vi "Modbus_FSM_Power_Dependence_Control.vi"() -> ()   [LabVIEW 2021]
uses:
  <vilib>/Plasmionique/MB Master/MB_Master/MB_Master.lvclass
  <vilib>/Plasmionique/MB Master/MB_Master_Serial/MB_Master_Serial.lvclass
  <vilib>/Plasmionique/MB Master/MB Master.lvlib
  <vilib>/Plasmionique/MB Master/MB_ADU/MB_ADU.lvclass
  C:/Program Files/National Instruments/LabVIEW 2021/vi.lib/Plasmionique/MB Master/MB_Master/MB_Master.lvclass
  Camera_Selected_g1.ctl
panel:
  in  "Direction Pulsed":bool
  in  "Total Scan Steps":i32(slide)=1 min=0 max=650000 step=10 scale=1.0..400000.0
  in  "Move Stage":bool
  in  "Scan g(1)":bool
  in  "Direction Stage":bool
  in  "Camera Selected":T1
  out "Scan Segments":i32
  out "Initial Segments":u16=10214
  in  "Steps":i32(slide)=1 min=0 max=650000 step=10 scale=1.0..400000.0
  out "Full Excitation Scan?":bool=TRUE
  out "Current Excitation HWP Segments":u8=230
  out "Initial Excitation QWP Segments":u8
  out "Current Excitation\nQWP angle":sgl
  in  "Event Registration Refnum":refnum<event-registration>
  in  "stop":bool
  out "Reset Modbus?":bool=TRUE
  in  "Modbus Address":refnum<visa-resource-name>="COM21"
  in  "Pulsed Power":dbl(slide)=1.0 min=0.0 max=180.0 step=0.001 scale=0.0..180.0
  in  "Scan Angle \nCW HWP":dbl=45.0
  in  "Etalon Angle":dbl(slide)=1.0 min=0.0 max=180.0 step=0.001 scale=0.0..180.0
  in  "CW Power":dbl(slide)=1.0 min=0.0 max=180.0 step=0.1 scale=0.0..180.0
  in  "Scan Angle\nPulsed HWP":dbl=45.0
  out "Def Pos CH3":u16[](array[numeric])
  out "Def Pos CH2":u16[](array[numeric])
  out "Def Pos CH1":u16[](array[numeric])
  out "Def Pos CH0":u16[](array[numeric])
  in  "Direction Etalon":bool
  in  "Direction CW":bool
  out "CH1 Steps/deg":u16=400
  out "CH0 Steps/deg":u16=400
  out "Current Collection HWP Segments":u8
  out "Initial Pulsed Segments":u8=230
  out "CH2 Steps/deg":u16=400
  out "CH3 Steps/deg":u16=400
  out "Current CW Segments":u8
  out "Initial Collection QWP Segments":u8=230
  out "Current CW angle":sgl
  out "Current Pulsed angle":sgl
  out "Full Collection Scan?":bool=TRUE
  out "Current Pulsed Segments":u8
  out "Initial CW Segments":u8=230
  out "Current Excitation\nHWP angle":sgl
  out "Def Pos CH0 Ind":bool=TRUE
  out "Def Pos CH1 Ind":bool=TRUE
  out "Def Pos CH2 Ind":bool=TRUE
  out "Def Pos CH3 Ind":bool=TRUE
  out "Pulsed?":bool=TRUE
  out "Last RX":string
  out "Last TX":string
  out "Last RX Time":string
  out "dt (ms)":u32=4
  out "Open?":bool
  out "Last Error Time":string
  out "Last Error Status":errorcluster
  in  "Reset Motor":bool
  in  "Rotate Etalon":bool
  in  "CW Power Rotate":bool
  in  "Pulsed Power Rotate":bool
  in  "Absolute Move CH0":bool=TRUE caption="Move to Default"
  in  "Absolute Move CH1":bool=TRUE
  in  "Absolute Move CH2":bool=TRUE
  in  "Absolute Move CH3":bool=TRUE
  in  "Set CH0 Default Position":bool=TRUE caption="Set Default"
  in  "Set CH1 Default Position":bool=TRUE
  in  "Set CH2 Default Position":bool=TRUE
  in  "Set CH3 Default Position":bool=TRUE
  in  "Power Dependence - CW":bool
  in  "Power Dependence - Pulsed":bool
  # "Power"
  # "Power Dependence"
  # "Direction"
  # "Rotate"
  # "g(1)"
  # "Direction"
  # "Etalon"
  # "Direction"
  # "Rotate"
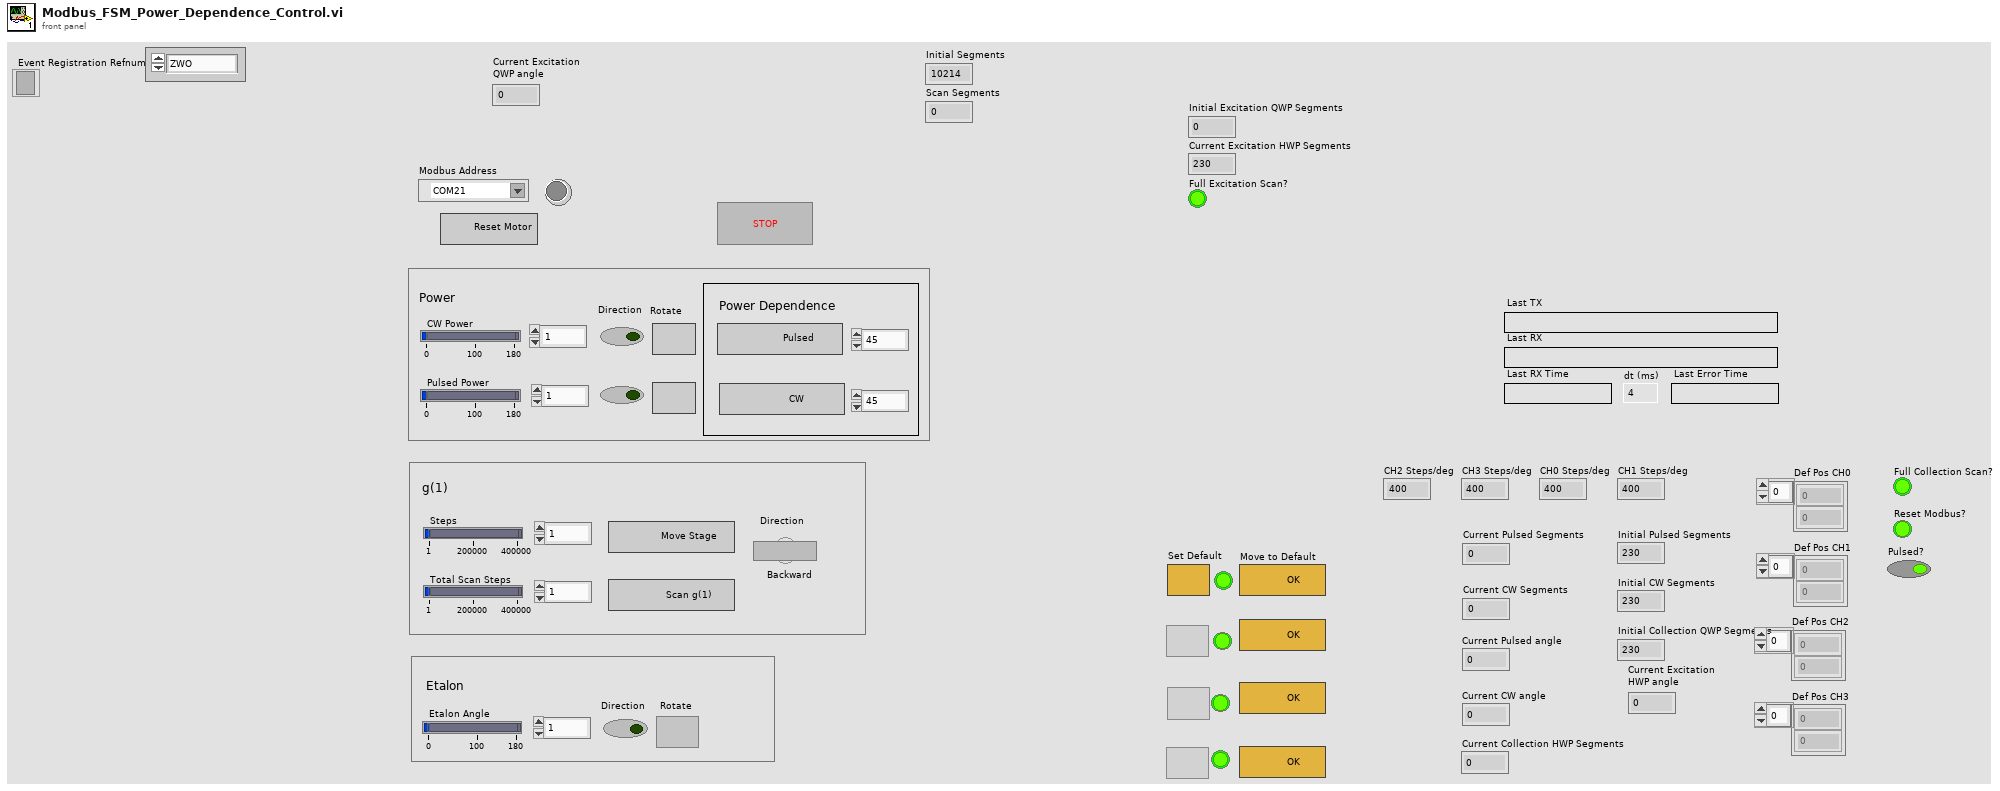
[diagram p1: front panel]
types:
  T1 = typedef "Camera_Selected_g1.ctl" = enum16{"ZWO", "qcmos"}
  T2 = cluster{"baud rate (bps)":u32, "stop bits":u16, "parity":u16, "flow control":u16, "timeout":u32, "retries":i32}
  T3 = enum8{"Enabled", "Disabled", "Disabled and Grayed Out"}
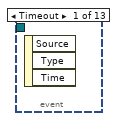
[diagram p2: hidden frame]
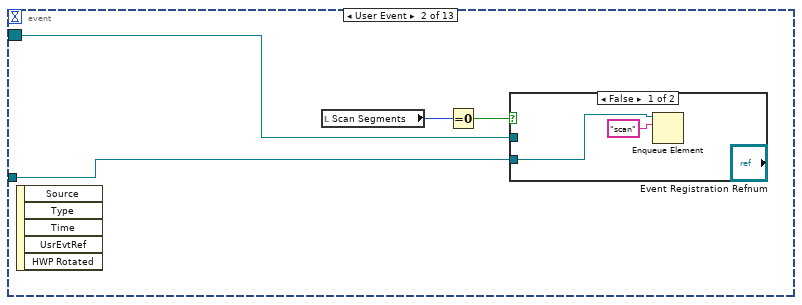
[diagram p3: hidden frame]
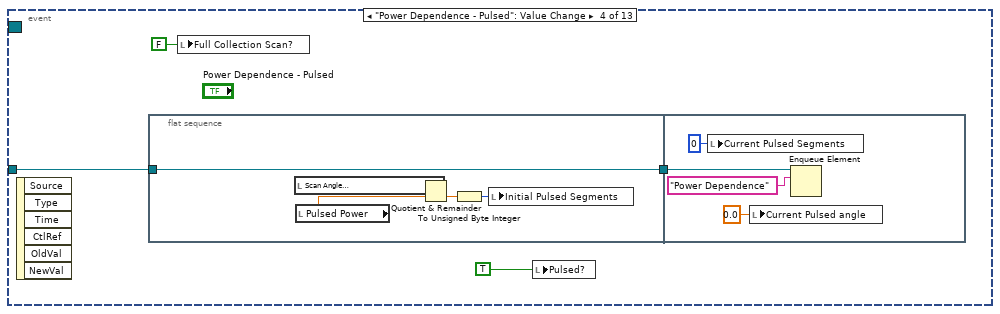
[diagram p5: hidden frame]
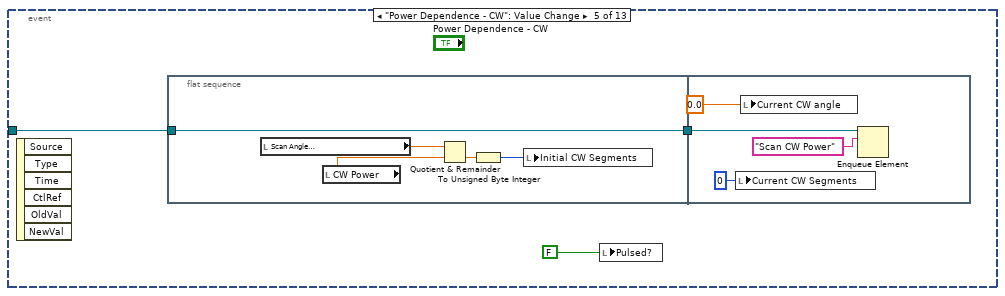
[diagram p6: hidden frame]
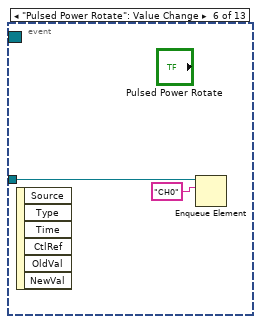
[diagram p7: hidden frame]
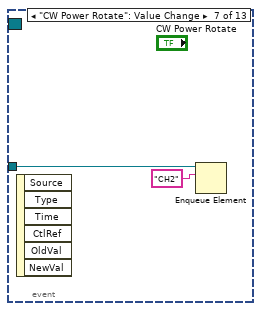
[diagram p8: hidden frame]
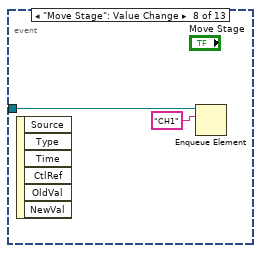
[diagram p9: hidden frame]
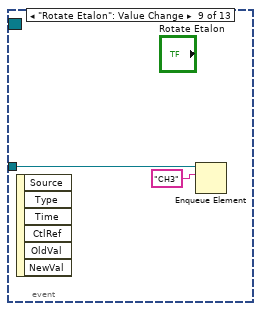
[diagram p10: hidden frame]
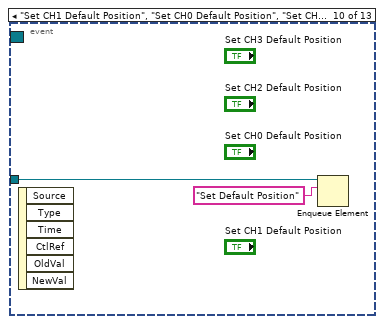
[diagram p11: hidden frame]
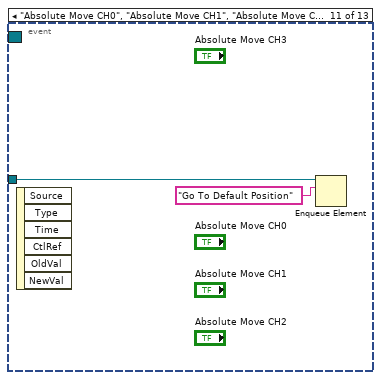
[diagram p12: hidden frame]
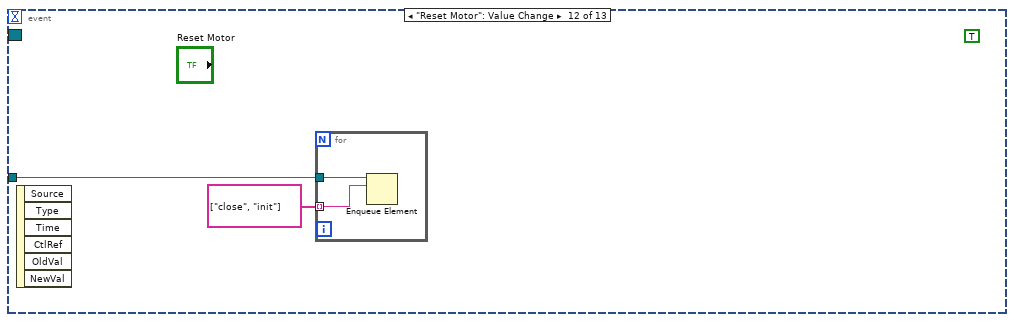
[diagram p13: hidden frame]
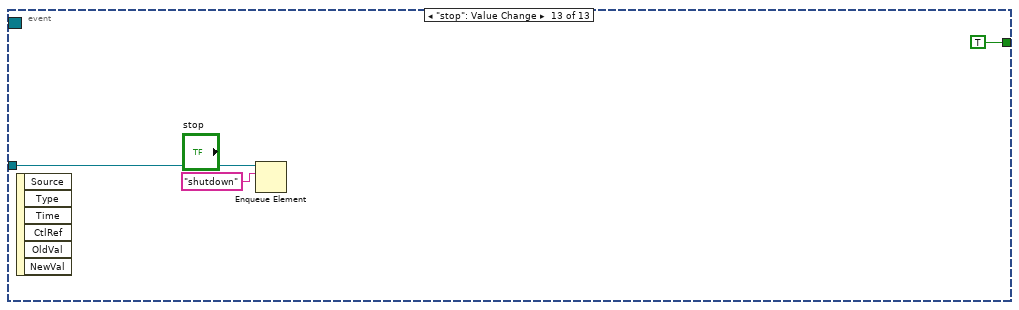
[diagram p14: hidden frame]
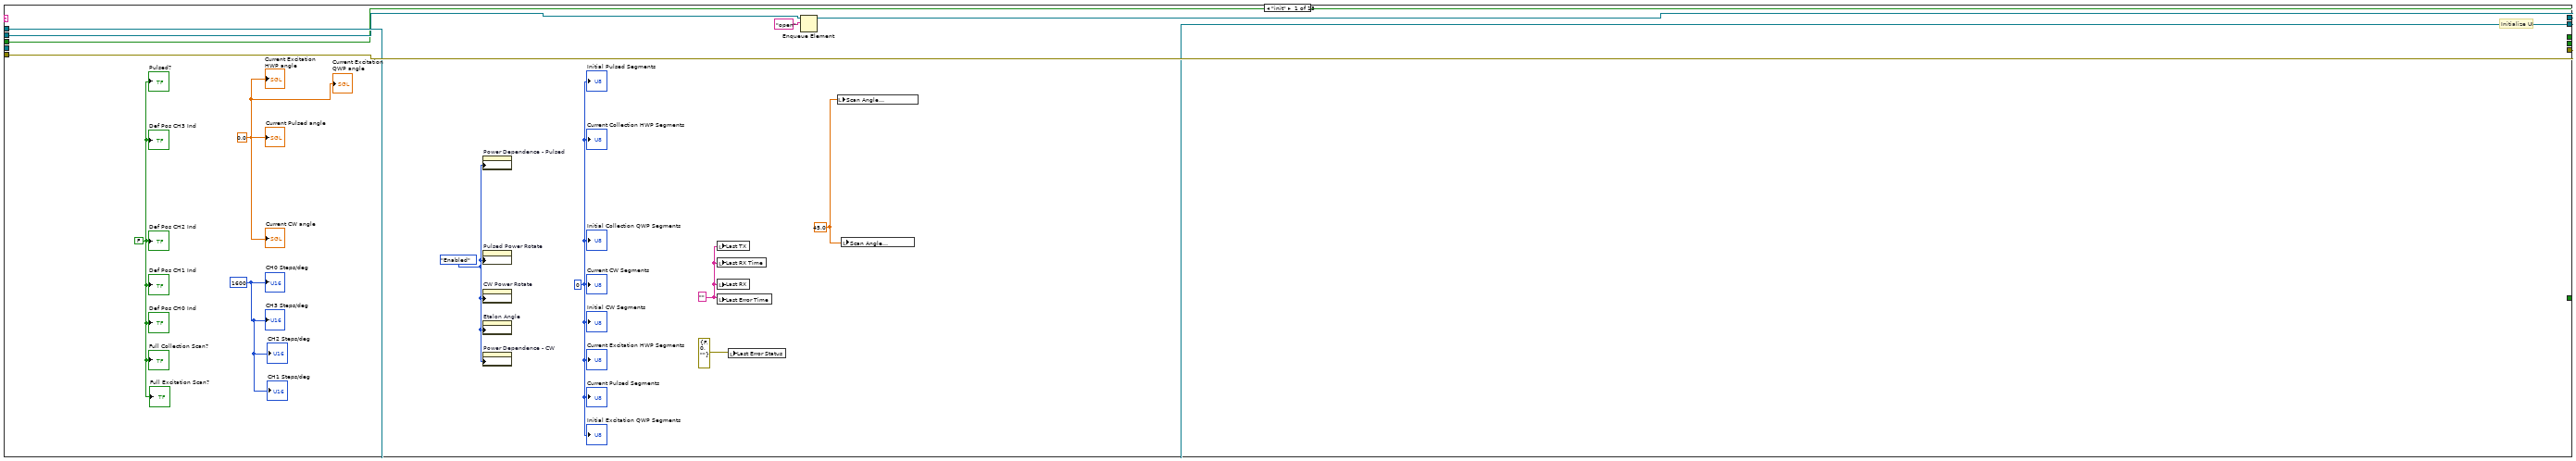
[diagram p17: hidden frame]
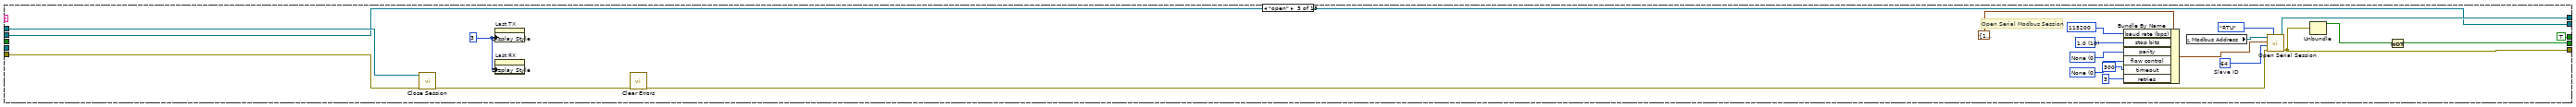
[diagram p18: hidden frame]
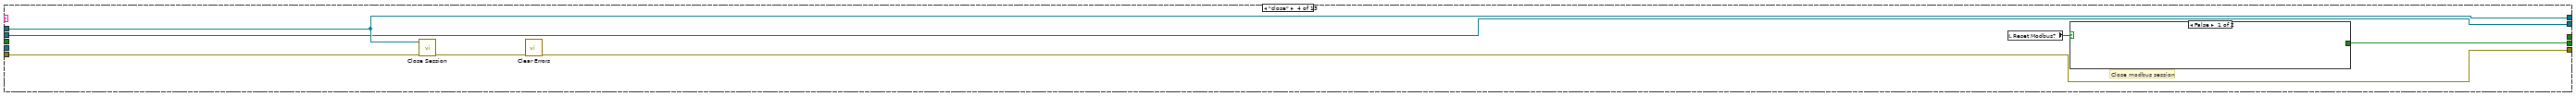
[diagram p19: hidden frame]
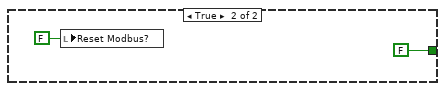
[diagram p20: hidden frame]
diagram:
  w1 = refnum<event-registration> refnum  # Event Registration Refnum
  w2 = refnum<user-event> refnum  # user event out
  n1 = Obtain Queue(element data type="") -> (queue out=w6:refnum<queue>)  [unwired: 4 in, 2 out]
  n2 = Enqueue Element(queue=w6, element="init") -> (queue out=w3:refnum<queue>)  [unwired: 2 in, 2 out]
  n3 = while {
    tunnel: w3 -> [w9]
    tunnel: w1 -> [w7]
    stop <- w8 stop-if-true
    # "UI Event Handler"
    n4 = event shown="[2] \"Scan g(1)\": Value Change" {
      selector: w7 -> [_ w11 _ _ _ _ _ _ _ _ _ _ _]
      dyn-events: _ -> [_ _ _ _ _ _ _ _ _ _ _ _ _]
      timeout: _ -> [_ _ _ _ _ _ _ _ _ _ _ _ _]
      tunnel: w9 -> [_ w10 w16 w25 w37 w48 w50 w52 w54 w55 w57 w60 w63]
      tunnel: [_ _ _ _ _ _ _ _ _ _ _ _ TRUE] -> w8
      event Timeout {
        n5 = event-data() -> ()  [unwired: 1 in, 3 out]
      }
      event User Event {
        n6 = event-data() -> ()  [unwired: 1 in, 5 out]
        n7 = local read "Scan Segments"() -> (w13:i32)
        n8 = Equal To 0?(x=w13) -> (x = 0?=w12:bool)
        n9 = case shown="False" w12 {
          tunnel: w11 -> [_ _]
          tunnel: w10 -> [w14 _]
          frame False {
            n10 = Enqueue Element(queue=w14, element="scan") -> ()  [unwired: 2 in, 3 out]
          }
          frame True {
          }
        }
      }
      event "Scan g(1)": Value Change {
        n11 = event-data() -> ()  [unwired: 1 in, 6 out]
        n12 = flat-sequence {
          tunnel: w16 -> [w20]
          frame #0 {
            n13 = local read "Total Scan Steps"() -> (w17:i32)
            n14 = local read "Steps"() -> (w18:i32)
            n15 = Quotient & Remainder(x=w17, y=w18) -> (floor(x/y)=w19:i32)  [unwired: 1 out]
            n16 = local write "Initial Segments"(w19) -> ()
            n17 = local write "Scan Segments"(w19) -> ()
          }
          frame #1 {
            n18 = Enqueue Element(queue=w20, element="scan") -> ()  [unwired: 2 in, 3 out]
          }
        }
      }
      event "Power Dependence - Pulsed": Value Change {
        n19 = event-data() -> ()  [unwired: 1 in, 6 out]
        n20 = flat-sequence {
          tunnel: w25 -> [w30]
          tunnel: [w30] -> w24
          tunnel: w24 -> [w33]
          frame #0 {
            n21 = local read "Scan Angle\nPulsed HWP"() -> (w26:dbl)
            n22 = local read "Pulsed Power"() -> (w29:dbl)
            n23 = Quotient & Remainder(x=w26, y=w29) -> (floor(x/y)=w28:dbl)  [unwired: 1 out]
            n24 = To Unsigned Byte Integer(number=w28) -> (unsigned 8bit integer=w27:u8)
            n25 = local write "Initial Pulsed Segments"(w27) -> ()
          }
          frame #1 {
            n26 = local write "Current Pulsed Segments"(u8 0 ("Current HWP Segmen")) -> ()
            n27 = local write "Current Pulsed angle"(sgl 0.0 ("Current Pulsed angle")) -> ()
            n28 = Enqueue Element(queue=w33, element="Power Dependence") -> ()  [unwired: 2 in, 3 out]
          }
        }
        n29 = local write "Full Collection Scan?"(FALSE ("Full Collection Scan?")) -> ()
        n30 = local write "Pulsed?"(TRUE ("Power Dependence?")) -> ()
      }
      event "Power Dependence - CW": Value Change {
        n31 = event-data() -> ()  [unwired: 1 in, 6 out]
        n32 = flat-sequence {
          tunnel: w37 -> [w42]
          tunnel: [w42] -> w36
          tunnel: w36 -> [w45]
          frame #0 {
            n33 = local read "Scan Angle\nPulsed HWP"() -> (w38:dbl)
            n34 = local read "CW Power"() -> (w41:dbl)
            n35 = Quotient & Remainder(x=w38, y=w41) -> (floor(x/y)=w40:dbl)  [unwired: 1 out]
            n36 = To Unsigned Byte Integer(number=w40) -> (unsigned 8bit integer=w39:u8)
            n37 = local write "Initial CW Segments"(w39) -> ()
          }
          frame #1 {
            n38 = local write "Current CW Segments"(u8 0 ("Current CW Segments")) -> ()
            n39 = local write "Current CW angle"(sgl 0.0 ("Current Excitation\nHWP angle")) -> ()
            n40 = Enqueue Element(queue=w45, element="Scan CW Power") -> ()  [unwired: 2 in, 3 out]
          }
        }
        n41 = local write "Pulsed?"(FALSE ("Power Dependence?")) -> ()
      }
      event "Pulsed Power Rotate": Value Change {
        n42 = event-data() -> ()  [unwired: 1 in, 6 out]
        n43 = Enqueue Element(queue=w48, element="CH0") -> ()  [unwired: 2 in, 3 out]
      }
      event "CW Power Rotate": Value Change {
        n44 = event-data() -> ()  [unwired: 1 in, 6 out]
        n45 = Enqueue Element(queue=w50, element="CH2") -> ()  [unwired: 2 in, 3 out]
      }
      event "Move Stage": Value Change {
        n46 = event-data() -> ()  [unwired: 1 in, 6 out]
        n47 = Enqueue Element(queue=w52, element="CH1") -> ()  [unwired: 2 in, 3 out]
      }
      event "Rotate Etalon": Value Change {
        n48 = event-data() -> ()  [unwired: 1 in, 6 out]
        n49 = Enqueue Element(queue=w54, element="CH3") -> ()  [unwired: 2 in, 3 out]
      }
      event "Set CH1 Default Position", "Set CH0 Default Position", "Set CH2 Default Position", "Set CH3 Default Position": Value Change {
        n50 = event-data() -> ()  [unwired: 1 in, 6 out]
        n51 = Enqueue Element(queue=w55, element="Set Default Position") -> ()  [unwired: 2 in, 3 out]
      }
      event "Absolute Move CH0", "Absolute Move CH1", "Absolute Move CH2", "Absolute Move CH3": Value Change {
        n52 = event-data() -> ()  [unwired: 1 in, 6 out]
        n53 = Enqueue Element(queue=w57, element="Go To Default Position") -> ()  [unwired: 2 in, 3 out]
      }
      event "Reset Motor": Value Change {
        (unwired) TRUE
        n54 = event-data() -> ()  [unwired: 1 in, 6 out]
        n55 = for {
          tunnel: w60 -> [w62]
          tunnel: string[] ["close", "init"] ("element") -> [w61] mode=indexing
          n56 = Enqueue Element(queue=w62, element=w61) -> ()  [unwired: 2 in, 3 out]
        }
      }
      event "stop": Value Change {
        n57 = event-data() -> ()  [unwired: 1 in, 6 out]
        n58 = Enqueue Element(queue=w63, element="shutdown") -> ()  [unwired: 2 in, 3 out]
      }
    }
  }
  n59 = while {
    tunnel: w3 -> [w77]
    shift-right: [w82] -> _
    shift-left: _ -> [w91]
    shift-right: [w87] -> _
    shift-left: _ -> [w88]
    tunnel: [w75] -> _
    shift-right: [w69] -> _
    shift-left: _ -> [w72]
    tunnel: w2 -> [w66]
    stop <- w70 stop-if-true
    w89 = 100  # Poll Period (ms)
    # "COMM Handler"
    n60 = Get Queue Status(queue=w77) -> (queue out=w76:refnum<queue>)  [unwired: 2 in, 7 out]
    n61 = Dequeue Element(queue=w76, timeout in ms (-1)=w89) -> (queue out=w90:refnum<queue>, element=w85:string, timed out?=w86:bool)  [unwired: 1 in, 1 out]
    n62 = flat-sequence {
      tunnel: [w109] -> w73
      tunnel: w86 -> [w108]
      tunnel: w85 -> [w107]
      tunnel: [w105] -> w84
      frame #0 {
        n63 = Tick Count (ms)() -> (millisecond timer value=w109:u32)
        n64 = Select(t="poll", s=w108, f=w107) -> (s? t:f=w105:string)
      }
    }
    n65 = case shown="\"shutdown\", Default" w84 {
      tunnel: [w141 w148 w173 w177 w185 w187 w209 w225 w241 w267 w322 w355 w407] -> w74
      tunnel: w91 -> [w141 w148 w170 w177 w185 w189 w208 w224 w240 w263 w324 w357 w414]
      tunnel: [w143 w149 w172 w178 w186 w192 w210 w226 w242 w271 w320 w356 w410] -> w81
      tunnel: w88 -> [w143 w151 w169 w180 w186 w194 w211 w227 w243 w265 w325 w364 w415]
      tunnel: [w138 FALSE ("EXIT") w166 w174 w183 w188 w207 w223 w239 w269 _ w354 w406] -> w68
      tunnel: w90 -> [w140 w147 w160 w175 w184 w196 w212 w228 w244 w270 w321 w362 w409]
      tunnel: [w139 w147 w160 w175 w184 w196 w212 w228 w244 w270 w321 w362 w409] -> w78
      tunnel: w66 -> [_ _ _ _ _ _ _ _ _ w273 w323 _ _]
      tunnel: w72 -> [w138 _ _ _ w183 w188 w207 w223 w239 w269 w319 w354 w406]
      tunnel: [_ _ TRUE _ _ w188 w207 w223 w239 w269 w319 w354 w406] -> w71
      tunnel: [_ TRUE _ _ _ _ _ _ _ _ _ _ _] -> w70
      frame "init" {
        w131 = FALSE ("Def Pos CH2 Ind")
        w132 = 45.0 ("Scan Angle \nHWP")
        w134 = sgl 0.0 ("Current HWP angle")
        w136 = T3."Enabled" ("Disabled")
        w133 = 0 ("floor(x/y)")
        w135 = u16 1600 ("Etalon Steps/deg")
        w142 = "" ("Last Error Time")
        # "Initialize UI"
        n66 = property on="Power Dependence - Pulsed" class="Bool"("DisabledEnum"=w136) -> ()  [unwired: 2 in, 2 out]
        n67 = property on="Pulsed Power Rotate" class="Bool"("DisabledEnum"=w136) -> ()  [unwired: 2 in, 2 out]
        n68 = property on="CW Power Rotate" class="Bool"("DisabledEnum"=w136) -> ()  [unwired: 2 in, 2 out]
        n69 = property on="Etalon Angle" class="Slide (strict)"("DisabledEnum"=w136) -> ()  [unwired: 2 in, 2 out]
        n70 = property on="Power Dependence - CW" class="Bool"("DisabledEnum"=w136) -> ()  [unwired: 2 in, 2 out]
        n71 = local write "Last TX"(w142) -> ()
        n72 = local write "Last RX Time"(w142) -> ()
        n73 = local write "Last RX"(w142) -> ()
        n74 = local write "Last Error Time"(w142) -> ()
        n75 = local write "Last Error Status"(errorcluster {"status"=FALSE, "code"=0, "source"=""} ("Last Error Status")) -> ()
        n76 = Enqueue Element(queue=w140, element="open") -> (queue out=w139:refnum<queue>)  [unwired: 2 in, 2 out]
        n77 = local write "Scan Angle\nPulsed HWP"(w132) -> ()
        n78 = local write "Scan Angle \nCW HWP"(w132) -> ()
        "CH1 Steps/deg" <- w135
        "CH0 Steps/deg" <- w135
        "Current Collection HWP Segments" <- w133
        "Initial Pulsed Segments" <- w133
        "CH2 Steps/deg" <- w135
        "CH3 Steps/deg" <- w135
        "Current CW Segments" <- w133
        "Initial Collection QWP Segments" <- w133
        "Current CW angle" <- w134
        "Current Pulsed angle" <- w134
        "Full Collection Scan?" <- w131
        "Current Pulsed Segments" <- w133
        "Initial CW Segments" <- w133
        "Current Excitation\nHWP angle" <- w134
        "Def Pos CH0 Ind" <- w131
        "Def Pos CH1 Ind" <- w131
        "Def Pos CH2 Ind" <- w131
        "Def Pos CH3 Ind" <- w131
        "Pulsed?" <- w131
        "Current Excitation\nQWP angle" <- w134
        "Initial Excitation QWP Segments" <- w133
        "Current Excitation HWP Segments" <- w133
        "Full Excitation Scan?" <- w131
      }
      frame "shutdown", Default {
        # "Close modbus session on shutdown"
        n79 = call-dynamic "Close Session.vi"("error in (no error)"=w151, "MB session in"=w148) -> ("error out"=w150:errorcluster)  [unwired: 9 in]
        n80 = call <vilib>:"Clear Errors.vi"("error in (no error)"=w150) -> ("error out"=w149:errorcluster)  [unwired: 5 in, 1 out]
      }
      frame "open" {
        w154 = u32 115200 items=["9600"=9600, "19200"=19200, "38400"=38400, "57600"=57600, "115200"=115200, "460800"=460800, "921600"=921600] ("Baud Rate (bps)")
        w155 = u16 10 items=["1.0"=10, "1.5"=15, "2.0"=20] ("Stop Bits")
        w156 = u16 0 items=["None", "Odd", "Even", "Mark", "Space"] ("Parity")
        w157 = u16 0 items=["None", "XON/XOFF", "RTS/CTS", "XON/XOFF & RTS/CTS", "DTR/DSR", "XON/XOFF & DTR/DSR"] ("Flow Control")
        w161 = u8 64  # Slave ID
        w164 = u32 3 ("Display Style")
        # "Open Serial Modbus Session"
        n81 = call-dynamic "Close Session.vi"("error in (no error)"=w169, "MB session in"=w170) -> ("error out"=w171:errorcluster)  [unwired: 9 in]
        n82 = property on="Last TX" class="Str"("Display Style"=w164) -> ()  [unwired: 2 in, 2 out]
        n83 = property on="Last RX" class="Str"("Display Style"=w164) -> ()  [unwired: 2 in, 2 out]
        n84 = call <vilib>:"Clear Errors.vi"("error in (no error)"=w171) -> ("error out"=w168:errorcluster)  [unwired: 5 in, 1 out]
        n85 = Bundle By Name(cluster=T2 {"baud rate (bps)"=19200, "stop bits"=10, "parity"=0, "flow control"=0, "timeout"=1000, "retries"=1} ("Serial Config"), "baud rate (bps)"=w154, "stop bits"=w155, "parity"=w156, "flow control"=w157, "timeout"=u32 300 ("Timeout (ms)"), "retries"=3 ("Retries")) -> (w152:T2)
        n86 = local read "Modbus Address"() -> (w163:refnum<visa-resource-name>)
        n87 = call <vilib>:"Open Serial Session.vi"("Mode (RTU)"=enum16{"RTU", "ASCII"}."RTU", "Error in"=w168, "Slave ID"=w161, "Serial Config"=w152, "VISA Resource"=w163) -> ("Error out"=w172:errorcluster, "MB_Serial session"=w173:refnum<class "MB_Master_Serial.lvclass">)  [unwired: 5 in]
        n88 = Unbundle(w172) -> ("status"=w165:bool)  [unwired: 2 out]
        n89 = Not(x=w165) -> (.not. x?=w166:bool)
      }
      frame "close" {
        # "Close modbus session"
        n90 = call-dynamic "Close Session.vi"("error in (no error)"=w180, "MB session in"=w177) -> ("error out"=w179:errorcluster)  [unwired: 9 in]
        n91 = call <vilib>:"Clear Errors.vi"("error in (no error)"=w179) -> ("error out"=w178:errorcluster)  [unwired: 5 in, 1 out]
        n92 = local read "Reset Modbus?"() -> (w176:bool)
        n93 = case shown="False" w176 {
          tunnel: [_ FALSE ("stop")] -> w174
          frame False {
          }
          frame True {
            n94 = local write "Reset Modbus?"(FALSE ("Reset Modbus?")) -> ()
          }
        }
      }
      frame "poll" {
        # "Enqueue commands for polled data"
      }
      frame "CH0" {
        n95 = property on="Pulsed Power Rotate" class="Bool"(error in=w194, "DisabledEnum"=T3."Disabled and Grayed Out" ("Disabled")) -> (error out=w191:errorcluster)  [unwired: 1 in, 1 out]
        n96 = case shown="True" w188 {
          tunnel: w189 -> [w197 w206]
          tunnel: w191 -> [w198 w205]
          tunnel: [w198 w204] -> w190
          tunnel: [w197 w203] -> w187
          frame False {
          }
          frame True {
            n97 = local read "Direction Pulsed"() -> (w199:bool)
            n98 = local read "Pulsed Power"() -> (w202:dbl)
            n99 = local read "CH0 Steps/deg"() -> (w201:u16)
            n100 = call "CH0_Move.vi"("Direction"=w199, "Channel"=u8 0, "error in (no error)"=w205, "CH0 Steps/deg"=w201, "Collection HWP Angle"=w202, "MB_Master in"=w206) -> ("error out"=w204:errorcluster, "MB_Master out"=w203:refnum<class "MB_Master.lvclass">)  [unwired: 4 in]
          }
        }
        n101 = property on="Pulsed Power Rotate" class="Bool"(error in=w190, "DisabledEnum"=T3."Enabled" ("Disabled")) -> (error out=w192:errorcluster)  [unwired: 1 in, 1 out]
      }
      frame "CH1" {
        n102 = case shown="True" w207 {
          tunnel: w208 -> [w213 w222]
          tunnel: w211 -> [w214 w221]
          tunnel: [w214 w220] -> w210
          tunnel: [w213 w219] -> w209
          frame False {
          }
          frame True {
            n103 = local read "Direction Stage"() -> (w215:bool)
            n104 = local read "CH1 Steps/deg"() -> (w217:u16)
            n105 = local read "Steps"() -> (w218:i32)
            n106 = call "CH0_Move.vi"("Direction"=w215, "Channel"=u8 1, "error in (no error)"=w221, "CH0 Steps/deg"=w217, "Collection HWP Angle"=w218, "MB_Master in"=w222) -> ("error out"=w220:errorcluster, "MB_Master out"=w219:refnum<class "MB_Master.lvclass">)  [unwired: 4 in]
          }
        }
      }
      frame "CH2" {
        n107 = case shown="True" w223 {
          tunnel: w224 -> [w229 w238]
          tunnel: w227 -> [w230 w237]
          tunnel: [w230 w236] -> w226
          tunnel: [w229 w235] -> w225
          frame False {
          }
          frame True {
            n108 = local read "CH2 Steps/deg"() -> (w234:u16)
            n109 = local read "Direction CW"() -> (w232:bool)
            n110 = local read "CW Power"() -> (w231:dbl)
            n111 = call "CH0_Move.vi"("Direction"=w232, "Channel"=u8 2, "error in (no error)"=w237, "CH0 Steps/deg"=w234, "Collection HWP Angle"=w231, "MB_Master in"=w238) -> ("error out"=w236:errorcluster, "MB_Master out"=w235:refnum<class "MB_Master.lvclass">)  [unwired: 4 in]
          }
        }
      }
      frame "CH3" {
        n112 = case shown="True" w239 {
          tunnel: w240 -> [w245 w254]
          tunnel: w243 -> [w246 w253]
          tunnel: [w246 w252] -> w242
          tunnel: [w245 w251] -> w241
          frame False {
          }
          frame True {
            n113 = local read "Direction Etalon"() -> (w247:bool)
            n114 = local read "Etalon Angle"() -> (w250:dbl)
            n115 = local read "CH3 Steps/deg"() -> (w249:u16)
            n116 = call "CH0_Move.vi"("Direction"=w247, "Channel"=u8 3, "error in (no error)"=w253, "CH0 Steps/deg"=w249, "Collection HWP Angle"=w250, "MB_Master in"=w254) -> ("error out"=w252:errorcluster, "MB_Master out"=w251:refnum<class "MB_Master.lvclass">)  [unwired: 4 in]
          }
        }
      }
      frame "Power Dependence" {
        w256 = T3."Disabled and Grayed Out" ("Disabled")
        n117 = property on="Power Dependence - CW" class="Bool"("DisabledEnum"=w256) -> ()  [unwired: 2 in, 2 out]
        n118 = property on="Power Dependence - Pulsed" class="Bool"("DisabledEnum"=w256) -> ()  [unwired: 2 in, 2 out]
        n119 = property on="Etalon Angle" class="Slide (strict)"("DisabledEnum"=w256) -> ()  [unwired: 2 in, 2 out]
        n120 = property on="Pulsed Power Rotate" class="Bool"("DisabledEnum"=w256) -> ()  [unwired: 2 in, 2 out]
        n121 = property on="CW Power Rotate" class="Bool"("DisabledEnum"=w256) -> ()  [unwired: 2 in, 2 out]
        n122 = local read "Pulsed?"() -> (w255:bool)
        n123 = case shown="False" w255 {
          tunnel: [w276 w281] -> w266
          tunnel: [w275 w280] -> w261
          tunnel: [w274 w279] -> w258
          frame True {
            n124 = local read "Current Pulsed Segments"() -> (w276:u8)
            n125 = local read "Initial Pulsed Segments"() -> (w277:u8)
            n126 = local read "Pulsed Power"() -> (w275:dbl)
            n127 = Greater?(x=w277, y=w276) -> (0:w274:bool)
            n128 = Multiply(x=w276, y=w275) -> (x*y=w278:dbl)
            n129 = local write "Current Pulsed Segments"(w278) -> ()
          }
          frame False {
            n130 = local read "Current CW Segments"() -> (w281:u8)
            n131 = local read "Initial CW Segments"() -> (w282:u8)
            n132 = local read "CW Power"() -> (w280:dbl)
            n133 = Greater?(x=w282, y=w281) -> (0:w279:bool)
            n134 = Multiply(x=w281, y=w280) -> (x*y=w283:dbl)
            n135 = local write "Current CW Segments"(w283) -> ()
          }
        }
        n136 = Not(x=w258) -> (.not. x?=w257:bool)
        n137 = Equal To 0?(x=w266) -> (x = 0?=w260:bool)
        n138 = Or(x=w257, y=w260) -> (x .or. y?=w259:bool)
        n139 = case shown="False" w259 {
          tunnel: w265 -> [w293 w303]
          tunnel: [w288 w303] -> w264
          tunnel: w263 -> [w294 w302]
          tunnel: [w286 w302] -> w262
          tunnel: w261 -> [w292 _]
          tunnel: w255 -> [w284 _]
          frame False {
            n140 = case shown="True" w284 {
              tunnel: [w297 w299] -> w291
              tunnel: [w296 w298] -> w290
              tunnel: [u8 2 ("Channel") u8 0 ("Channel")] -> w285
              frame False {
                n141 = local read "CH2 Steps/deg"() -> (w297:u16)
                n142 = local read "Direction CW"() -> (w296:bool)
              }
              frame True {
                n143 = local read "CH0 Steps/deg"() -> (w299:u16)
                n144 = local read "Direction CW"() -> (w298:bool)
              }
            }
            n145 = call "CH0_Move.vi"("Direction"=w290, "Channel"=w285, "error in (no error)"=w293, "CH0 Steps/deg"=w291, "Collection HWP Angle"=w292, "MB_Master in"=w294) -> ("error out"=w289:errorcluster, "MB_Master out"=w287:refnum<class "MB_Master.lvclass">)  [unwired: 4 in]
            n146 = call "Modbus_Scan_Test.vi"("error in (no error)"=w289, "channel"=w285, "MB_Master in"=w287) -> ("error out"=w288:errorcluster, "MB_Master out"=w286:refnum<class "MB_Master.lvclass">)  [unwired: 7 in]
          }
          frame True {
            n147 = Wait (ms)(milliseconds to wait=u32 1000 ("Count(Ticks)")) -> ()  [unwired: 1 out]
          }
        }
        n148 = case shown="False" w258 {
          tunnel: ["Last Move" ("t") w316] -> w272
          tunnel: w260 -> [_ w313]
          tunnel: w264 -> [w306 w311]
          tunnel: w262 -> [w305 w312]
          tunnel: [w306 w311] -> w268
          tunnel: [w305 w312] -> w267
          tunnel: w266 -> [_ w310]
          frame False {
            w304 = T3."Enabled" ("Disabled")
            n149 = property on="Etalon Angle" class="Slide (strict)"("DisabledEnum"=w304) -> ()  [unwired: 2 in, 2 out]
            n150 = property on="Power Dependence - CW" class="Bool"("DisabledEnum"=w304) -> ()  [unwired: 2 in, 2 out]
            n151 = property on="Pulsed Power Rotate" class="Bool"("DisabledEnum"=w304) -> ()  [unwired: 2 in, 2 out]
            n152 = property on="Power Dependence - Pulsed" class="Bool"("DisabledEnum"=w304) -> ()  [unwired: 2 in, 2 out]
            n153 = property on="CW Power Rotate" class="Bool"("DisabledEnum"=w304) -> ()  [unwired: 2 in, 2 out]
          }
          frame True {
            n154 = local read "Pulsed?"() -> (w309:bool)
            n155 = Increment(x=w310) -> (x+1=w308:u8)
            n156 = case shown="False" w309 {
              tunnel: w308 -> [w317 w318]
              frame False {
                n157 = local write "Current CW Segments"(w317) -> ()
              }
              frame True {
                n158 = local write "Current Pulsed Segments"(w318) -> ()
              }
            }
            n159 = Select(t="First Scan", s=w313, f="") -> (s? t:f=w316:string)
          }
        }
        n160 = Generate User Event(user event=w273, event data cluster=w272, error in=w268) -> (error out=w271:errorcluster)  [unwired: 1 in, 1 out]
      }
      frame "g(1) scan" {
        w328 = u16 3 ("CH0 Steps/deg")
        n161 = local read "Direction Stage"() -> (w332:bool)
        n162 = local read "Initial Segments"() -> (w336:u16)
        n163 = local read "Scan Segments"() -> (w334:i32)
        n164 = local read "Steps"() -> (w333:i32)
        n165 = Equal?(x=w334, y=w336) -> (x = y?=w335:bool)
        n166 = call "CH0_Move.vi"("Direction"=w332, "Channel"=w328, "error in (no error)"=w325, "CH0 Steps/deg"=u16 1, "Collection HWP Angle"=w333, "MB_Master in"=w324) -> ("error out"=w330:errorcluster, "MB_Master out"=w331:refnum<class "MB_Master.lvclass">)  [unwired: 4 in]
        n167 = Decrement(x=w334) -> (x-1=w337:i32)
        n168 = Greater?(x=w334, y=1) -> (0:w340:bool)
        n169 = local write "Scan Segments"(w337) -> ()
        n170 = case shown="True" w340 {
          tunnel: ["Last Move" w352] -> w339
          tunnel: w335 -> [_ w353]
          frame False {
          }
          frame True {
            n171 = Select(t="First Scan", s=w353, f="") -> (s? t:f=w352:string)
          }
        }
        n172 = call "Modbus_Scan_Test.vi"("error in (no error)"=w330, "channel"=w328, "MB_Master in"=w331) -> ("error out"=w329:errorcluster, "MB_Master out"=w322:refnum<class "MB_Master.lvclass">)  [unwired: 7 in]
        n173 = local read "Camera Selected"() -> (w338:T1)
        n174 = case shown="\"ZWO\", Default" w338 {
          tunnel: [w343 w348] -> w320
          tunnel: w329 -> [w341 w347]
          tunnel: w323 -> [w342 w346]
          tunnel: w339 -> [_ w345]
          frame "ZWO" {
            n175 = Generate User Event(user event=w342, event data cluster="self.start_acquisition()", error in=w341) -> (error out=w343:errorcluster)  [unwired: 1 in, 1 out]
          }
          frame "ZWO", Default {
            n176 = Generate User Event(user event=w346, event data cluster=w345, error in=w347) -> (error out=w348:errorcluster)  [unwired: 1 in, 1 out]
          }
        }
      }
      frame "Go To Default Position" {
        n177 = local read "Absolute Move CH0"() -> (w375:bool)
        n178 = local read "Absolute Move CH1"() -> (w374:bool)
        n179 = local read "Absolute Move CH2"() -> (w373:bool)
        n180 = local read "Absolute Move CH3"() -> (w372:bool)
        n181 = case shown="True" w375 {
          tunnel: [_ "CH0"] -> w371
          frame False {
          }
          frame True {
            n182 = local write "Absolute Move CH0"(FALSE ("Get CH0 Default Position")) -> ()
          }
        }
        n183 = case shown="True" w374 {
          tunnel: [_ "CH1"] -> w370
          frame False {
          }
          frame True {
            n184 = local write "Absolute Move CH1"(FALSE ("Get CH0 Default Position")) -> ()
          }
        }
        n185 = case shown="True" w373 {
          tunnel: [_ "CH2"] -> w369
          frame False {
          }
          frame True {
            n186 = local write "Absolute Move CH2"(FALSE ("Get CH0 Default Position")) -> ()
          }
        }
        n187 = case shown="True" w372 {
          tunnel: [_ "CH3"] -> w368
          frame False {
          }
          frame True {
            n188 = local write "Absolute Move CH3"(FALSE ("Get CH0 Default Position")) -> ()
          }
        }
        n189 = Concatenate Strings(w371, w370, w369, w368) -> (w363:string)
        n190 = case shown="\"CH0\"" w363 {
          tunnel: w364 -> [_ w388 w391 w394 w397]
          tunnel: [errorcluster {"status"=TRUE, "code"=0, "source"="Absolute Position Movement \nAbs Move CH ERROR"} ("error out") w388 w391 w394 w397] -> w358
          tunnel: [_ w387 w390 w392 w396] -> w359
          tunnel: [999 0 ("y") 1 ("x") 2 ("x") 3 ("x")] -> w361
          frame "False", Default {
          }
          frame "CH0" {
            n191 = local read "Def Pos CH0"() -> (w387:u16[])
          }
          frame "CH1" {
            n192 = local read "Def Pos CH1"() -> (w390:u16[])
          }
          frame "CH2" {
            n193 = local read "Def Pos CH0"() -> (w392:u16[])
          }
          frame "CH3" {
            n194 = local read "Def Pos CH3"() -> (w396:u16[])
          }
        }
        n195 = Multiply(x=w361, y=100) -> (x*y=w365:i32)
        n196 = Add(x=10116, y=w365) -> (x+y=w360:i32)
        n197 = case shown="True" w354 {
          tunnel: w357 -> [w377 w383]
          tunnel: w360 -> [_ w382]
          tunnel: w358 -> [w376 w381]
          tunnel: w359 -> [_ w378]
          tunnel: [w377 w380] -> w355
          tunnel: [w376 w379] -> w356
          frame False {
          }
          frame True {
            n198 = call <vilib>:"Write Multiple Registers.vi"("error in (no error)"=w381, "values"=w378, "starting address"=w382, "MB session in"=w383) -> ("error out"=w379:errorcluster, "MB session out"=w380:refnum<class "MB_Master.lvclass">)  [unwired: 6 in]
          }
        }
      }
      frame "Set Default Position" {
        n199 = local read "Set CH0 Default Position"() -> (w428:bool)
        n200 = local read "Set CH1 Default Position"() -> (w427:bool)
        n201 = local read "Set CH2 Default Position"() -> (w426:bool)
        n202 = local read "Set CH3 Default Position"() -> (w425:bool)
        n203 = case shown="True" w428 {
          tunnel: [_ "Get CH0 Default Position"] -> w424
          frame False {
          }
          frame True {
            n204 = local write "Set CH0 Default Position"(FALSE ("Get CH0 Default Position")) -> ()
          }
        }
        n205 = case shown="True" w427 {
          tunnel: [_ "Get CH1 Default Position"] -> w423
          frame False {
          }
          frame True {
            n206 = local write "Set CH1 Default Position"(FALSE ("Get CH0 Default Position")) -> ()
          }
        }
        n207 = case shown="True" w426 {
          tunnel: [_ "Get CH2 Default Position"] -> w422
          frame False {
          }
          frame True {
            n208 = local write "Set CH2 Default Position"(FALSE ("Get CH0 Default Position")) -> ()
          }
        }
        n209 = case shown="True" w425 {
          tunnel: [_ "Get CH3 Default Position"] -> w421
          frame False {
          }
          frame True {
            n210 = local write "Set CH3 Default Position"(FALSE ("Get CH0 Default Position")) -> ()
          }
        }
        n211 = Concatenate Strings(w424, w423, w422, w421) -> (w413:string)
        n212 = case shown="\"False\", Default" w413 {
          tunnel: [999 0 1 2 3] -> w408
          tunnel: w415 -> [_ w456 w458 w460 w462]
          tunnel: [errorcluster {"status"=TRUE, "code"=0, "source"=""} ("error out 2") w456 w458 w460 w462] -> w416
          frame "False", Default {
          }
          frame "Get CH0 Default Position" {
          }
          frame "Get CH1 Default Position" {
          }
          frame "Get CH2 Default Position" {
          }
          frame "Get CH3 Default Position" {
          }
        }
        n213 = Multiply(x=w408, y=100) -> (x*y=w418:i32)
        n214 = Add(x=10102, y=w418) -> (x+y=w417:i32)
        n215 = case shown="True" w406 {
          tunnel: w414 -> [w446 w453]
          tunnel: w417 -> [_ w452]
          tunnel: w416 -> [w445 w450]
          tunnel: [w445 w449] -> w411
          tunnel: [w446 w448] -> w407
          tunnel: [w443 w447] -> w412
          frame False {
            n216 = Build Array(u16 0, u16 0 ("element")) -> (w443:u16[])
          }
          frame True {
            n217 = call <vilib>:"Read Holding Registers.vi"("error in (no error)"=w450, "quantity"=u16 2, "starting address"=w452, "MB session in"=w453) -> ("error out"=w449:errorcluster, "Registers"=w447:u16[], "MB session out"=w448:refnum<class "MB_Master.lvclass">)  [unwired: 5 in]
          }
        }
        n218 = case shown="\"False\", Default" w413 {
          tunnel: w412 -> [_ w432 w435 w438 w441]
          tunnel: w411 -> [w429 w431 w434 w437 w440]
          tunnel: [w429 w431 w434 w437 w440] -> w410
          frame "False", Default {
          }
          frame "Get CH0 Default Position" {
            n219 = local write "Def Pos CH0 Ind"(TRUE ("Def Pos CH0 Ind")) -> ()
            "Def Pos CH0" <- w432
          }
          frame "Get CH1 Default Position" {
            n220 = local write "Def Pos CH1 Ind"(TRUE ("Def Pos CH0 Ind")) -> ()
            "Def Pos CH1" <- w435
          }
          frame "Get CH2 Default Position" {
            n221 = local write "Def Pos CH2 Ind"(TRUE ("Def Pos CH0 Ind")) -> ()
            "Def Pos CH2" <- w438
          }
          frame "Get CH3 Default Position" {
            n222 = local write "Def Pos CH3 Ind"(TRUE ("Def Pos CH0 Ind")) -> ()
            "Def Pos CH3" <- w441
          }
        }
      }
    }
    n223 = case shown="True" w71 {
      tunnel: w74 -> [w113 w117]
      tunnel: [w113 w128] -> w83
      tunnel: w73 -> [_ w122]
      tunnel: w81 -> [w112 w116]
      tunnel: [w112 w115] -> w80
      tunnel: w78 -> [w111 w118]
      tunnel: [w111 w118] -> w79
      tunnel: w68 -> [w110 w114]
      tunnel: [w110 w114] -> w67
      frame False {
      }
      frame True {
        n224 = property class="MB_Master"(reference=w117, error in=w116) -> (reference out=w128:refnum<class "MB_Master.lvclass">, error out=w115:errorcluster, "Properties:ADU"=w129:refnum<class "MB_ADU.lvclass">)
        n225 = Tick Count (ms)() -> (millisecond timer value=w121:u32)
        n226 = local write "Last Error Time"("" ("Last Error Time")) -> ()
        n227 = local write "Last Error Status"(errorcluster {"status"=FALSE, "code"=0, "source"=""} ("Last Error Status")) -> ()
        n228 = property class="MB_ADU"(reference=w129) -> ("Properties:TX Data"=→"Last TX":string, "Properties:RX Data"=→"Last RX":string, "Properties:RX Timestamp"=w119:timestamp)  [unwired: 1 in, 2 out]
        n229 = Subtract(x=w121, y=w122) -> (x-y=→"dt (ms)":u32)
        n230 = Format Date/Time String(time format string (%c)="%H:%M:%S%3u", seconds (now)=w119) -> (date/time string=→"Last RX Time":string)  [unwired: 1 in]
      }
    }
    n231 = case shown="Error" w80 {
      selector: w80 -> [w95 w97]
      tunnel: [w95 w101] -> w87
      tunnel: w79 -> [w94 w99]
      tunnel: [w94 w98] -> w75
      tunnel: w83 -> [w93 w96]
      tunnel: [w93 w96] -> w82
      tunnel: w67 -> [w92 _]
      tunnel: [w92 _] -> w69
      frame No Error {
      }
      frame Error {
        # "Clear error and close modbus session"
        n232 = Enqueue Element(queue=w99, element="close") -> (queue out=w98:refnum<queue>)  [unwired: 2 in, 2 out]
        n233 = Get Date/Time In Seconds() -> (seconds since 1Jan1904=w102:timestamp)
        n234 = Format Date/Time String(time format string (%c)="%H:%M:%S%3u", seconds (now)=w102) -> (date/time string=→"Last Error Time":string)  [unwired: 1 in]
        n235 = call <vilib>:"Clear Errors.vi"("error in (no error)"=w97) -> ("error out"=w101:errorcluster)  [unwired: 5 in, 1 out]
        "Last Error Status" <- w97
      }
    }
    "Open?" <- w72
  }
